vi "JSON Array to LabVIEW Array Base Type.vi"(8 "error in (no error)":errorcluster, 10 "Type of Array In":T1=enum."Unknown", 11 "JSON Array In":variant) -> (0 "error out":errorcluster, 3 "LabVIEW Array Base Type Out":variant)   [LabVIEW 2010, in "i3-json.lvlib"]
uses:
  i3-json.lvlib
  JSON Types/JSON Type.ctl
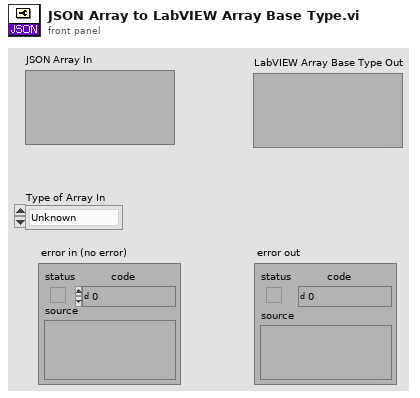
[diagram p1: front panel]
types:
  T1 = typedef "i3-json.lvlib/JSON Type.ctl" = enum8{"JSON Compatible", "JSON Array", "JSON Object", "JSON Null", "Double", "String", "Boolean", "Unknown"}
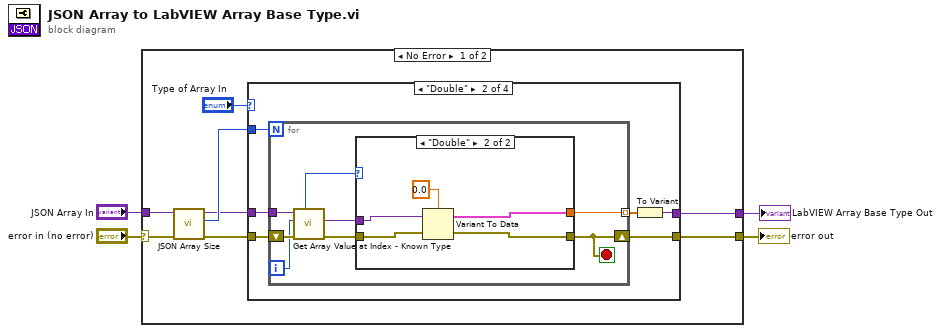
[diagram p0: block diagram]
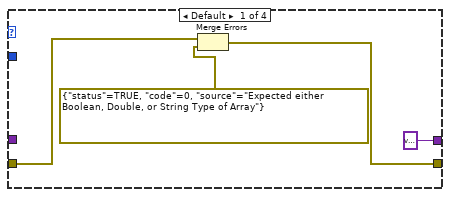
[diagram p2: hidden frame]
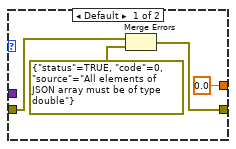
[diagram p3: hidden frame]
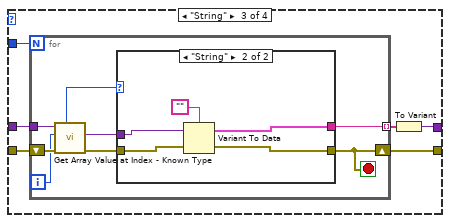
[diagram p4: hidden frame]
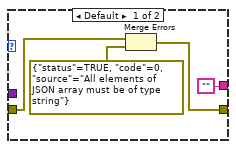
[diagram p5: hidden frame]
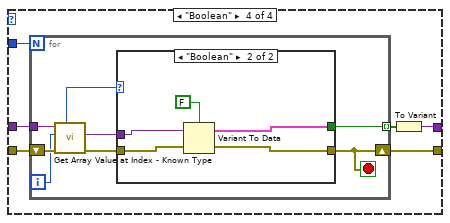
[diagram p6: hidden frame]
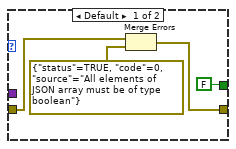
[diagram p7: hidden frame]
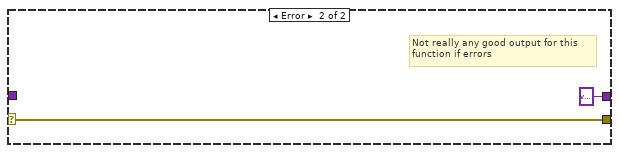
[diagram p8: hidden frame]
diagram:
  n1 = case shown="No Error" "error in (no error)" {
    selector: "error in (no error)" -> [w6 w86]
    tunnel: "JSON Array In" -> [w5 _]
    tunnel: [w12 w86] -> w2
    tunnel: [w11 variant ("Variant")] -> w1
    frame No Error {
      n2 = call "JSON Array Size.vi"("error in (no error)"=w6, "JSON Tree In (JSON Array)"=w5) -> ("error out"=w9:errorcluster, "Array Size"=w10:i32, "JSON Tree Passthrough (JSON Array)"=w8:variant)  [unwired: 7 in]
      n3 = case shown="\"Double\"" "Type of Array In" {
        tunnel: w10 -> [_ w22 w45 w68]
        tunnel: w9 -> [w14 w21 w44 w67]
        tunnel: w8 -> [_ w20 w43 w66]
        tunnel: [w15 w19 w42 w65] -> w12
        tunnel: [variant ("Variant") w18 w41 w64] -> w11
        frame Default {
          n4 = Merge Errors(w14, errorcluster {"status"=TRUE, "code"=0, "source"="Expected either Boolean, Double, or String Type of Array"} ("error in")) -> (w15:errorcluster)
        }
        frame "Double" {
          n5 = for {
            N: w22 -> [_]
            tunnel: w20 -> [w30]
            tunnel: [w24] -> w17 mode=indexing
            shift-right: [w23] -> w19
            shift-left: w21 -> [w29]
            i -> [w28]
            stop <- w23 stop-if-true
            n6 = call "Get Array Value at Index - Known Type.vi"("error in (no error)"=w29, "Index"=w28, "JSON Tree In (JSON Array)"=w30) -> ("error out"=w25:errorcluster, "Value"=w26:variant, "JSON Type"=w27:T1)  [unwired: 3 in, 3 out]
            n7 = case shown="\"Double\"" w27 {
              tunnel: w26 -> [_ w38]
              tunnel: w25 -> [w32 w39]
              tunnel: [w33 w36] -> w23
              tunnel: [0.0 w35] -> w24
              frame Default {
                n8 = Merge Errors(w32, errorcluster {"status"=TRUE, "code"=0, "source"="All elements of JSON array must be of type double"} ("error in")) -> (w33:errorcluster)
              }
              frame "Double" {
                n9 = Variant To Data(error in=w39, Variant=w38, type=0.0) -> (error out=w36:errorcluster, data=w35:cluster{})
              }
            }
          }
          n10 = To Variant(anything=w17) -> (Variant=w18:variant)
        }
        frame "String" {
          n11 = for {
            N: w45 -> [_]
            tunnel: w43 -> [w53]
            tunnel: [w47] -> w40 mode=indexing
            shift-right: [w46] -> w42
            shift-left: w44 -> [w52]
            i -> [w51]
            stop <- w46 stop-if-true
            n12 = call "Get Array Value at Index - Known Type.vi"("error in (no error)"=w52, "Index"=w51, "JSON Tree In (JSON Array)"=w53) -> ("error out"=w48:errorcluster, "Value"=w49:variant, "JSON Type"=w50:T1)  [unwired: 3 in, 3 out]
            n13 = case shown="\"String\"" w50 {
              tunnel: w49 -> [_ w61]
              tunnel: w48 -> [w56 w62]
              tunnel: [w57 w60] -> w46
              tunnel: ["" w59] -> w47
              frame Default {
                n14 = Merge Errors(w56, errorcluster {"status"=TRUE, "code"=0, "source"="All elements of JSON array must be of type string"} ("error in")) -> (w57:errorcluster)
              }
              frame "String" {
                n15 = Variant To Data(error in=w62, Variant=w61, type="") -> (error out=w60:errorcluster, data=w59:cluster{})
              }
            }
          }
          n16 = To Variant(anything=w40) -> (Variant=w41:variant)
        }
        frame "Boolean" {
          n17 = for {
            N: w68 -> [_]
            tunnel: w66 -> [w76]
            tunnel: [w70] -> w63 mode=indexing
            shift-right: [w69] -> w65
            shift-left: w67 -> [w75]
            i -> [w74]
            stop <- w69 stop-if-true
            n18 = call "Get Array Value at Index - Known Type.vi"("error in (no error)"=w75, "Index"=w74, "JSON Tree In (JSON Array)"=w76) -> ("error out"=w71:errorcluster, "Value"=w72:variant, "JSON Type"=w73:T1)  [unwired: 3 in, 3 out]
            n19 = case shown="\"Boolean\"" w73 {
              tunnel: w72 -> [_ w84]
              tunnel: w71 -> [w79 w85]
              tunnel: [w80 w83] -> w69
              tunnel: [FALSE w82] -> w70
              frame Default {
                n20 = Merge Errors(w79, errorcluster {"status"=TRUE, "code"=0, "source"="All elements of JSON array must be of type boolean"} ("error in")) -> (w80:errorcluster)
              }
              frame "Boolean" {
                n21 = Variant To Data(error in=w85, Variant=w84, type=FALSE) -> (error out=w83:errorcluster, data=w82:cluster{})
              }
            }
          }
          n22 = To Variant(anything=w63) -> (Variant=w64:variant)
        }
      }
    }
    frame Error {
      # "Not really any good output for this\nfunction if errors"
    }
  }
  "LabVIEW Array Base Type Out" <- w1
  "error out" <- w2
